vi "LimeLight targeting.vi"(7 "targetHeight (in)":dbl, 8 "error in (no error)":errorcluster, 11 "LIMELIGHT pose":T2={"Installed?"=FALSE, "pose"={"X"=0.0, "Y"=-3.0, "Z"=22.0, "angle to horizon"=-22.0, "tx angle offset"=0.0}}) -> (0 "error out":errorcluster, 1 "LOCK?":bool, 2 "DistanceToTarget":dbl=26.235051697949295, 3 "BRNG (deg)":dbl=-2.0)   [LabVIEW 2023]
uses:
  ctrl defs/ctrl LimeLight target.ctl
  ctrl defs/ctrl LIMELIGHT initialize.ctl
  <vilib>/Rock Robotics/Network Tables/NT Read Number.vi
  <vilib>/Rock Robotics/Network Tables/NT Read Integer.vi
  Global odometry.vi
  <vilib>/Rock Robotics/WPI/ThirdParty/JAS_Junk/TrajLib/Trajectory_Library.lvlib
panel:
  in  "Limelight target\ntest input":T1={"tv"=1, "tx"=-3.0, "ty"=-15.0, "ta"=0.8}
  in  "testing?":bool
  out "LimeLight\ntargeting data":T1={"tv"=1, "tx"=-3.0, "ty"=-15.0, "ta"=0.8}
  in  "stop":bool
  # "for TESTING loop only"
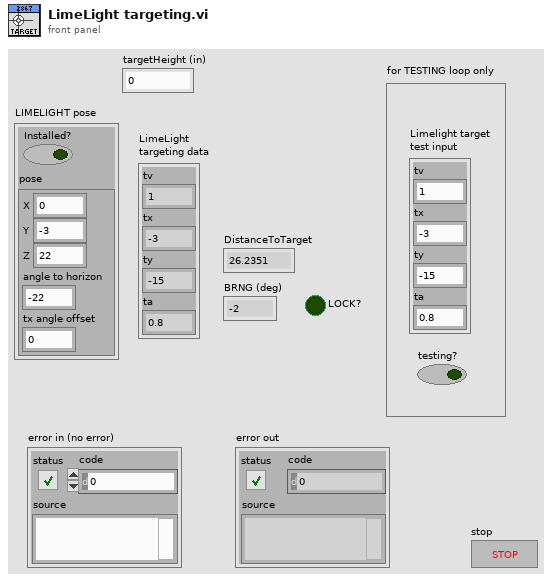
[diagram p1: front panel]
types:
  T1 = typedef "ctrl LimeLight target.ctl" = cluster{"tv":u8, "tx":dbl, "ty":dbl, "ta":dbl}
  T2 = typedef "ctrl LIMELIGHT initialize.ctl" = cluster{"Installed?":bool, "pose":cluster{"X":dbl, "Y":dbl, "Z":dbl, "angle to horizon":dbl, "tx angle offset":dbl}}
  T3 = cluster{"X":dbl, "Y":dbl, "Z":dbl, "angle to horizon":dbl, "tx angle offset":dbl}
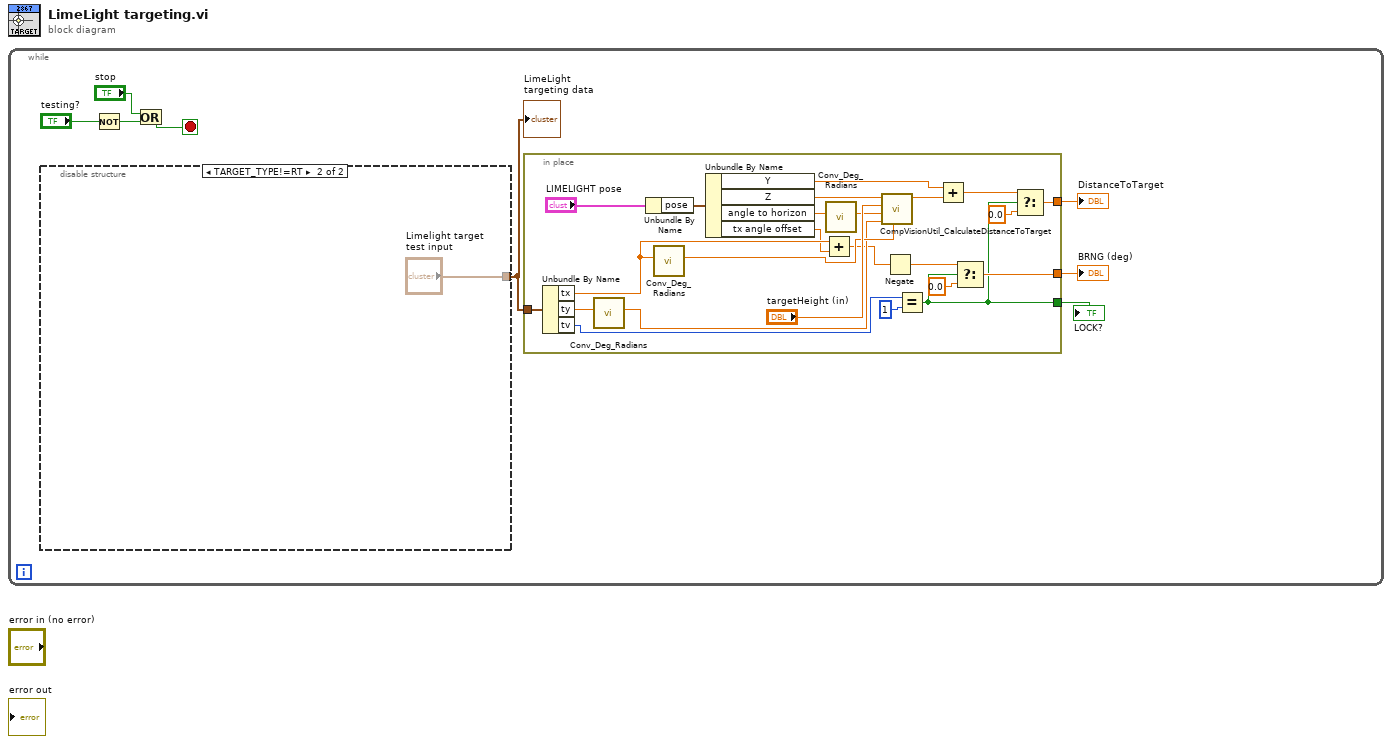
[diagram p0: block diagram]
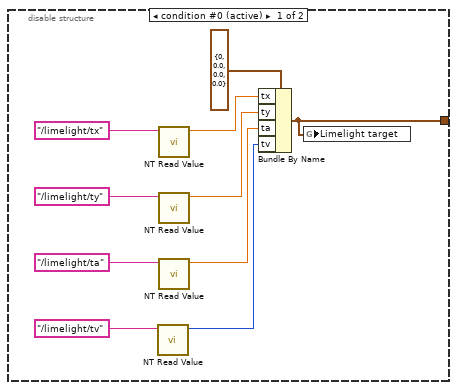
[diagram p2: hidden frame]
diagram:
  n1 = while {
    stop <- w6 stop-if-true
    n2 = disable-structure shown="TARGET_TYPE!=RT" {
      disable-tunnel: [w33 "Limelight target\ntest input"] -> w4
      frame condition #0 (active) {
        n3 = call-poly <vilib>:"NT Read Value.vi"("name"="/limelight/tv") -> ("value"=w34:i64)  [unwired: 8 in, 2 out]
        n4 = call-poly <vilib>:"NT Read Value.vi"("name"="/limelight/tx") -> ("value"=w37:dbl)  [unwired: 8 in, 2 out]
        n5 = call-poly <vilib>:"NT Read Value.vi"("name"="/limelight/ty") -> ("value"=w36:dbl)  [unwired: 8 in, 2 out]
        n6 = call-poly <vilib>:"NT Read Value.vi"("name"="/limelight/ta") -> ("value"=w35:dbl)  [unwired: 8 in, 2 out]
        n7 = Bundle By Name(cluster=T1 {"tv"=0, "tx"=0.0, "ty"=0.0, "ta"=0.0} ("Limelight target"), "tx"=w37, "ty"=w36, "ta"=w35, "tv"=w34) -> (w33:T1)
        n8 = global write "Global odometry.vi" "Limelight target"(w33) -> ()
      }
      frame condition #1 {
      }
    }
    "LimeLight\ntargeting data" <- w4
    n9 = Not(x="testing?") -> (.not. x?=w8:bool)
    n10 = Or(x="stop", y=w8) -> (x .or. y?=w6:bool)
    n11 = in-place {
      in-place-border: w4 -> [w30]
      in-place-border: [w17] -> w3
      in-place-border: [w16] -> w2
      in-place-border: [w9] -> w1
      n12 = Unbundle By Name(w30) -> ("tx"=w19:dbl, "ty"=w26:dbl, "tv"=w14:u8)
      n13 = call <vilib>:"Conv_Deg_Radians.vi"("Degress"=w26) -> ("Radians"=w24:dbl)  [unwired: 10 in]
      n14 = Unbundle By Name("LIMELIGHT pose") -> ("pose"=w31:T3)
      n15 = call <vilib>:"Conv_Deg_Radians.vi"("Degress"=w19) -> ("Radians"=w25:dbl)  [unwired: 10 in]
      n16 = Unbundle By Name(w31) -> ("Y"=w21:dbl, "Z"=w29:dbl, "angle to horizon"=w27:dbl, "tx angle offset"=w18:dbl)
      n17 = Add(x=w19, y=w18) -> (x+y=w15:dbl)
      n18 = call <vilib>:"Conv_Deg_Radians.vi"("Degress"=w27) -> ("Radians"=w23:dbl)  [unwired: 10 in]
      n19 = call <vilib>:"CompVisionUtil_CalculateDistanceToTarget.vi"("TargetYawRadians"=w25, "targetPitch_Radians"=w24, "cameraPitch_Radians"=w23, "targetHeight_Meters"="targetHeight (in)", "cameraHeight_Meters"=w29) -> ("DistanceToTarget_Meters"=w22:dbl)  [unwired: 6 in]
      n20 = Negate(x=w15) -> (-x=w10:dbl)
      n21 = Equal?(x=w14, y=u8 1) -> (x = y?=w9:bool)
      n22 = Add(x=w21, y=w22) -> (x+y=w20:dbl)
      n23 = Select(t=w10, s=w9, f=0.0) -> (s? t:f=w16:dbl)
      n24 = Select(t=w20, s=w9, f=0.0) -> (s? t:f=w17:dbl)
    }
    "DistanceToTarget" <- w3
    "BRNG (deg)" <- w2
    "LOCK?" <- w1
  }
